vi "Set diameter.vi"(7 "[x]":T1, 8 "error in (no error)":errorcluster, 10 "Diameter (mm)":dbl, 11 "Serial Port in":refnum<visa-resource-name>) -> (0 "error out":errorcluster, 3 "Serial Port out":refnum<visa-resource-name>)   [LabVIEW 2016, in "Chemyx_Syringe_Pump_driver.lvlib"]
doc: "Sets the diameter of the syringe in mm.\n\nInput diameter is a double float."
uses:
  Chemyx_Syringe_Pump_driver.lvlib
  _private/Control/Control Mode.ctl
panel:
  # "Sets the diameter of the syringe in mm.\n\nInput diameter is a double float."
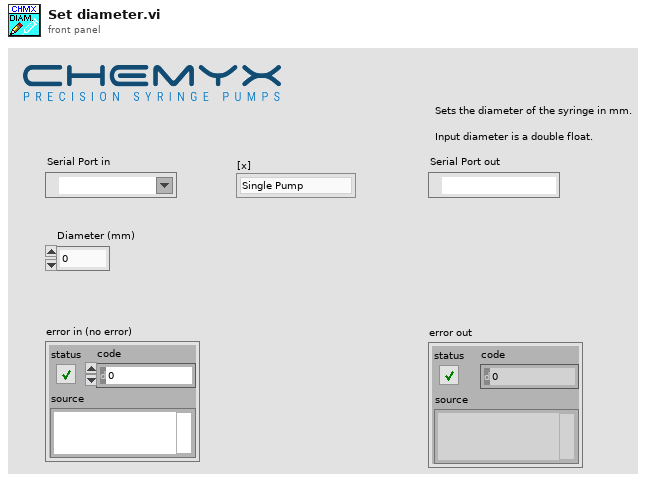
[diagram p1: front panel]
types:
  T1 = typedef "Chemyx_Syringe_Pump_driver.lvlib/Control Mode.ctl" = enum16{"Single Pump", "Pump Chanel 1", "Pump Channel 2", "Cycle Mode"}
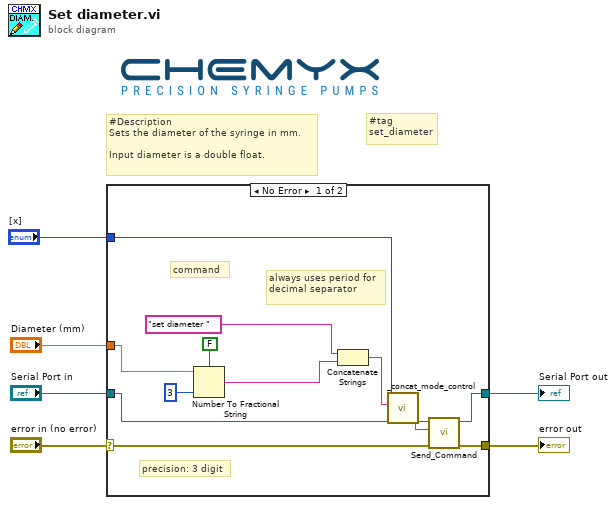
[diagram p0: block diagram]
diagram:
  # "#tag\nset_diameter"
  # "#Description\nSets the diameter of the syringe in mm.\n\nInput diameter is a double float."
  n1 = case shown="No Error" "error in (no error)" {
    selector: "error in (no error)" -> [w17 w20]
    tunnel: "Serial Port in" -> [w18 w19]
    tunnel: [w16 w20] -> w4
    tunnel: [w15 w19] -> w3
    tunnel: "Diameter (mm)" -> [w13 _]
    tunnel: "[x]" -> [w7 _]
    frame No Error {
      # "always uses period for decimal separator"
      # "precision: 3 digit"
      # "command"
      n2 = Number To Fractional String(use system decimal point (T)=FALSE, number=w13, precision (6)=i16 3) -> (F-format string=w11:string)  [unwired: 1 in]
      n3 = Concatenate Strings("set diameter ", w11) -> (w9:string)
      n4 = call "_concat_mode_control.vi"("write buffer"=w9, "[x]"=w7) -> ("write buffer out"=w8:string)  [unwired: 9 in]
      n5 = call "Send_Command.vi"("error in (no error)"=w17, "write buffer"=w8, "Serial Port in"=w18) -> ("error out"=w16:errorcluster, "VISA Refnum out"=w15:refnum<visa-resource-name>)  [unwired: 6 in, 1 out]
    }
    frame Error {
    }
  }
  "error out" <- w4
  "Serial Port out" <- w3
